vi "Start Module.vi"(6 "Show Main VI Diagram on Init (F)":bool, 8 "error in":errorcluster) -> (0 "error out":errorcluster, 1 "Wait for Event Sync?":bool, 2 "Panther Dashboard Broadcast Events":T1, 3 "Module Was Already Running?":bool)   [LabVIEW 2019, in "Panther Dashboard.lvlib"]
doc: "Launches the module Main VI. After calling this VI, you can optionally register for broadcast events from the module by wiring the broadcast events output of this VI to a <b>Register For Events</b> function. \n\nAfter the optional Register For Events function call, you should always call the <b>Synchronize Module Events.vi</b> for this module with the 'Wait for Event Sync?' output of this VI to the corresponding input of the Synchronize Module Events.vi. \n\nTo see an example of the proper wiring pattern, see the \"Start Module: Value Change\" event frame in the API Tester VI for this module.\n_____\nBased on DQMH Project Template 6.1.0.94."
uses:
  Panther Dashboard.lvlib
  Broadcast Events--cluster.ctl
  Did Init Argument--cluster.ctl
  Status Updated Argument--cluster.ctl
  Error Reported Argument--cluster.ctl
  Stop Argument--cluster.ctl
  Get Module Execution Status Argument--cluster.ctl
  References Updated Argument--cluster.ctl
  Module type--enum.ctl
  Projects Updated Argument--cluster.ctl
  Targets Updated Argument--cluster.ctl
  Progress updated Argument--cluster.ctl
  Scale Updated Argument--cluster.ctl
  Connector Pane Updated Argument--cluster.ctl
  Documentation Updated Argument--cluster.ctl
  Documentation--cluster.ctl
  Module Type Updated Argument--cluster.ctl
  Theme Updated Argument--cluster.ctl
  Project Description Updated Argument--cluster.ctl
  <vilib>/Delacor/Delacor QMH/Libraries/Module Admin_class/Delacor_lib_QMH_Module Admin.lvclass
  <vilib>/Delacor/Delacor QMH/Libraries/Module Admin_class/Delacor_lib_QMH_Module Admin.lvclass/Delacor_lib_QMH_Module Admin.ctl
  <vilib>/Delacor/Delacor QMH/Libraries/Module Admin_class/Delacor_lib_QMH_Set External Launch.vi
  <vilib>/Utility/error.llb/Error Cluster From Error Code.vi
  <vilib>/ErrorRing/Error Ring.xnode
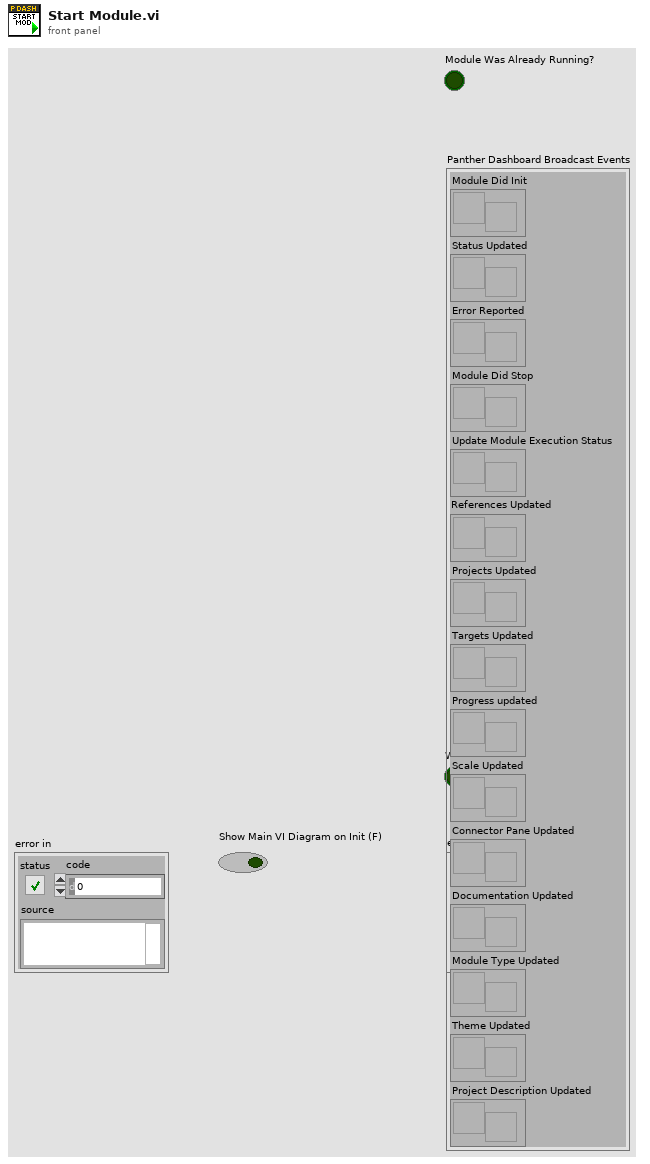
[diagram p1: front panel]
types:
  T1 = typedef "Panther Dashboard.lvlib/Broadcast Events--cluster.ctl" = cluster{"Module Did Init":refnum<user-event>, "Status Updated":refnum<user-event>, "Error Reported":refnum<user-event>, "Module Did Stop":refnum<user-event>, "Update Module Execution Status":refnum<user-event>, "References Updated":refnum<user-event>, "Projects Updated":refnum<user-event>, "Targets Updated":refnum<user-event>, "Progress updated":refnum<user-event>, "Scale Updated":refnum<user-event>, "Connector Pane Updated":refnum<user-event>, "Documentation Updated":refnum<user-event>, "Module Type Updated":refnum<user-event>, "Theme Updated":refnum<user-event>, "Project Description Updated":refnum<user-event>}
  T2 = enum32{"Bad", "Idle", "Run top level", "Running"}
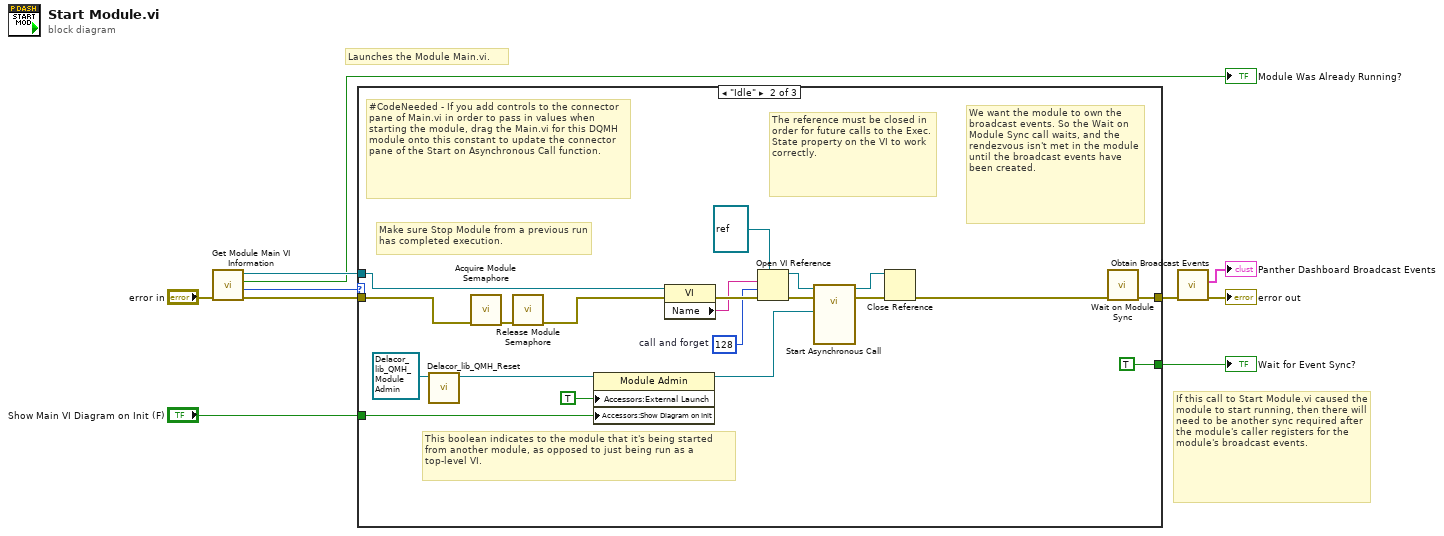
[diagram p0: block diagram]
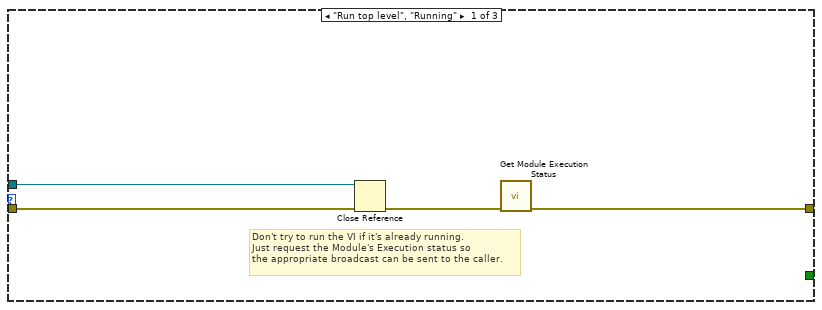
[diagram p2: hidden frame]
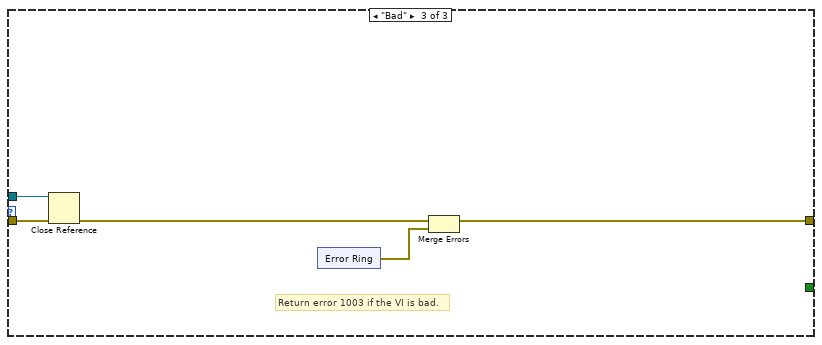
[diagram p3: hidden frame]
diagram:
  # "If this call to Start Module.vi caused the module to start running, then there will need to be another sync required after the module's caller registers for the module's broadcast events."
  # "Launches the Module Main.vi."
  n1 = call "Get Module Main VI Information.vi"("error in"="error in") -> ("error out"=w10:errorcluster, "Execution State"=w4:T2, "Is Module Running?"=→"Module Was Already Running?":bool, "Module Main VI"=w6:refnum<vi>)  [unwired: 7 in]
  n2 = case shown="\"Idle\"" w4 {
    tunnel: w10 -> [w14 w28 w39]
    tunnel: w6 -> [w11 w22 w35]
    tunnel: [w12 w34 w37] -> w9
    tunnel: [_ TRUE _] -> w5
    tunnel: "Show Main VI Diagram on Init (F)" -> [_ w15 _]
    frame "Run top level", "Running" {
      # "Don't try to run the VI if it's already running.\nJust request the Module's Execution status so\nthe appropriate broadcast can be sent to the caller."
      n3 = Close Reference(reference=w11, error in (no error)=w14) -> (error out=w13:errorcluster)
      n4 = call "Get Module Execution Status.vi"("error in (no error)"=w13) -> ("error out"=w12:errorcluster)  [unwired: 10 in]
    }
    frame "Idle" {
      w20 = 128  # call and forget
      # "Make sure Stop Module from a previous run has completed execution."
      # "#CodeNeeded - If you add controls to the connector pane of Main.vi in order to pass in values when starting the module, drag the Main.vi for this DQMH module onto this constant to update the connector pane of the Start on Asynchronous Call function."
      # "The reference must be closed in order for future calls to the Exec.State property on the VI to work correctly."
      # "We want the module to own the broadcast events. So the Wait on Module Sync call waits, and the rendezvous isn't met in the module until the broadcast events have been created."
      # "This boolean indicates to the module that it's being started from another module, as opposed to just being run as a top-level VI."
      n5 = call-dynamic "Delacor_lib_QMH_Reset.vi"("Mod Admin in"=refnum<class "Delacor_lib_QMH_Module Admin.lvclass"> refnum) -> ("Mod Admin out"=w25:refnum<class "Delacor_lib_QMH_Module Admin.lvclass">)  [unwired: 9 in, 1 out]
      n6 = call "Acquire Module Semaphore.vi"("error in"=w28) -> ("error out"=w29:errorcluster)  [unwired: 10 in]
      n7 = call "Release Module Semaphore.vi"("error in"=w29) -> ("error out"=w27:errorcluster)  [unwired: 10 in]
      n8 = property class="Module Admin"(reference=w25, "Accessors:External Launch"=TRUE, "Accessors:Show Diagram on Init"=w15) -> (reference out=w18:refnum<class "Delacor_lib_QMH_Module Admin.lvclass">)  [unwired: 1 in, 1 out]
      n9 = property class="VI"(reference=w22, error in=w27) -> (error out=w33:errorcluster, "Name"=w16:string)  [unwired: 1 out]
      n10 = Open VI Reference(type specifier VI Refnum (for type only)=refnum<vi> refnum, vi path=w16, options=w20, error in (no error)=w33) -> (vi reference=w19:refnum<vi>, error out=w32:errorcluster)  [unwired: 2 in]
      n11 = call-by-ref "Start Asynchronous Call"(reference=w19, error in=w32, "Module Admin"=w18) -> (reference out=w17:refnum<vi>, error out=w31:errorcluster)  [unwired: 11 in]
      n12 = Close Reference(reference=w17, error in (no error)=w31) -> (error out=w30:errorcluster)
      n13 = call "Wait on Module Sync.vi"("error in (no error)"=w30) -> ("error out"=w34:errorcluster)  [unwired: 10 in]
    }
    frame "Bad" {
      # "Return error 1003 if the VI is bad."
      n14 = Close Reference(reference=w35, error in (no error)=w39) -> (error out=w38:errorcluster)
      n15 = xnode "Error Ring"() -> ("error out"=w36:errorcluster)
      n16 = Merge Errors(w38, w36) -> (w37:errorcluster)
    }
  }
  "Wait for Event Sync?" <- w5
  n17 = call "Obtain Broadcast Events.vi"("error in"=w9) -> ("error out"=→"error out":errorcluster, "Panther Dashboard Broadcast Events"=→"Panther Dashboard Broadcast Events":T1)  [unwired: 9 in]
